vi "快捷菜单激活(表格).vi"(11 "菜单引用":refnum<k9>) -> ()   [LabVIEW 2021]
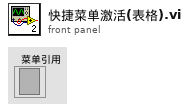
[diagram p1: front panel]
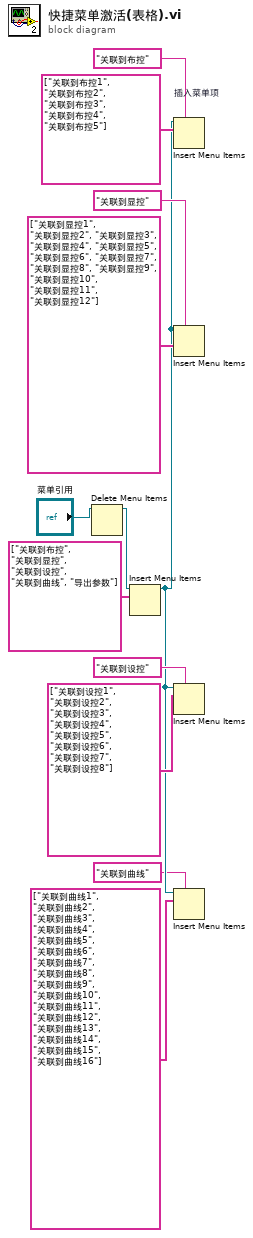
[diagram p0: block diagram]
diagram:
  n1 = Delete Menu Items(9:"菜单引用") -> (3:w12:refnum<k9>)  [unwired: 3 in, 1 out]
  n2 = Insert Menu Items ("插入菜单项")(8:string[] ["关联到布控", "关联到显控", "关联到设控", "关联到曲线", "导出参数"] ("项名称"), 9:w12) -> (3:w2:refnum<k9>)  [unwired: 4 in, 2 out]
  n3 = Insert Menu Items "插入菜单项"(5:"关联到布控" ("菜单标识符"), 8:string[] ["关联到布控1", "关联到布控2", "关联到布控3", "关联到布控4", "关联到布控5"] ("项名称"), 9:w2) -> ()  [unwired: 3 in, 3 out]
  n4 = Insert Menu Items ("插入菜单项")(5:"关联到显控" ("菜单标识符"), 7:string[] ["关联到显控1", "关联到显控2", "关联到显控3", "关联到显控4", "关联到显控5", "关联到显控6", "关联到显控7", "关联到显控8", "关联到显控9", "关联到显控10", "关联到显控11", "关联到显控12"] ("项标识符"), 9:w2) -> ()  [unwired: 3 in, 3 out]
  n5 = Insert Menu Items ("插入菜单项")(5:"关联到设控" ("菜单标识符"), 8:string[] ["关联到设控1", "关联到设控2", "关联到设控3", "关联到设控4", "关联到设控5", "关联到设控6", "关联到设控7", "关联到设控8"] ("项名称"), 9:w2) -> ()  [unwired: 3 in, 3 out]
  n6 = Insert Menu Items ("插入菜单项")(5:"关联到曲线" ("菜单标识符"), 8:string[] ["关联到曲线1", "关联到曲线2", "关联到曲线3", "关联到曲线4", "关联到曲线5", "关联到曲线6", "关联到曲线7", "关联到曲线8", "关联到曲线9", "关联到曲线10", "关联到曲线11", "关联到曲线12", "关联到曲线13", "关联到曲线14", "关联到曲线15", "关联到曲线16"] ("项名称"), 9:w2) -> ()  [unwired: 3 in, 3 out]
